vi "getModbus.vi"(11 "Mockbus in":refnum<class "Mockbus.lvclass">) -> (2 "Modbus.lvclass":refnum<class "Modbus.lvclass">, 3 "Mockbus out":refnum<class "Mockbus.lvclass">)   [LabVIEW 2015, in "Mockbus.lvclass"]
uses:
  Mockbus.lvclass
  Modbus/Modbus/Modbus.lvclass
  Mockbus.lvclass/Mockbus.ctl
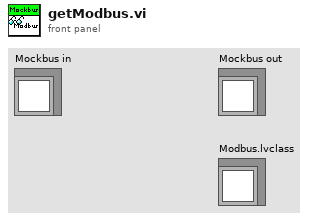
[diagram p1: front panel]
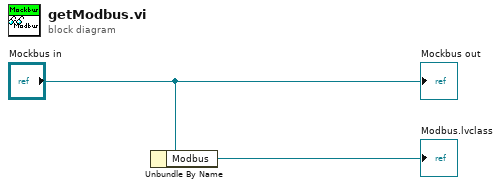
[diagram p0: block diagram]
diagram:
  n1 = Unbundle By Name("Mockbus in") -> ("Modbus"=→"Modbus.lvclass":refnum<class "Modbus.lvclass">)
  "Mockbus out" <- "Mockbus in"
